vi "lcm.vi"(2 "Values":i32[](array[numeric])) -> (0 "LCM":i32)   [LabVIEW 2018]
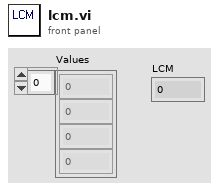
[diagram p1: front panel]
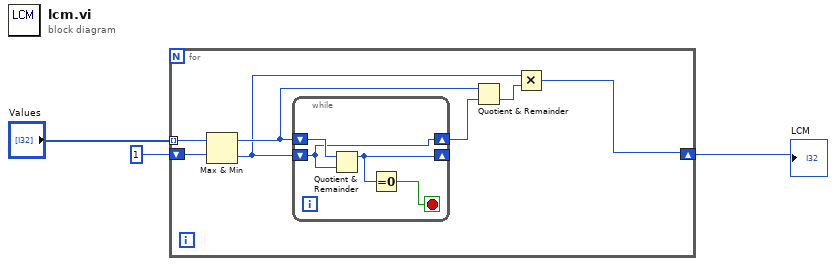
[diagram p0: block diagram]
diagram:
  n1 = for {
    tunnel: "Values" -> [w10] mode=indexing
    shift-right: [w4] -> w1
    shift-left: 1 -> [w5]
    n2 = Max & Min(x=w10, y=w5) -> (max(x,y)=w8:i32, min(x,y)=w6:i32)
    n3 = while {
      shift-right: [w11] -> w9
      shift-left: w8 -> [w14]
      shift-right: [w13] -> _
      shift-left: w6 -> [w11]
      stop <- w12 stop-if-true
      n4 = Quotient & Remainder(x=w14, y=w11) -> (x-y*floor(x/y)=w13:i32)  [unwired: 1 out]
      n5 = Equal To 0?(x=w13) -> (x = 0?=w12:bool)
    }
    n6 = Quotient & Remainder(x=w8, y=w9) -> (floor(x/y)=w7:i32)  [unwired: 1 out]
    n7 = Multiply(x=w6, y=w7) -> (x*y=w4:i32)
  }
  "LCM" <- w1
